vi "step_HAPS_Compressor.vi"(8 "error in":errorcluster) -> (0 "error out":errorcluster)   [LabVIEW 2020]
uses:
  <vilib>/AKKA/PROVEtech-RBS/PROVEtechRBS.lvlib
  <vilib>/AKKA/PROVEtech-RBS/SubVIs/Write (Signals Single-point).vi
  <vilib>/AKKA/PROVEtech-RBS/SubVIs/Read (Signals Single-point).vi
panel:
  out "receive unit":string[](array[string])
  out "pass":bool
  out "Array out":string[](array[string])
  out "receive signals":string[](array[string])
  out "sgl array":dbl[](array[numeric])
  out "send unit":string[](array[string])
  out "send values":string[](array[string])
  out "send signals":string[](array[string])
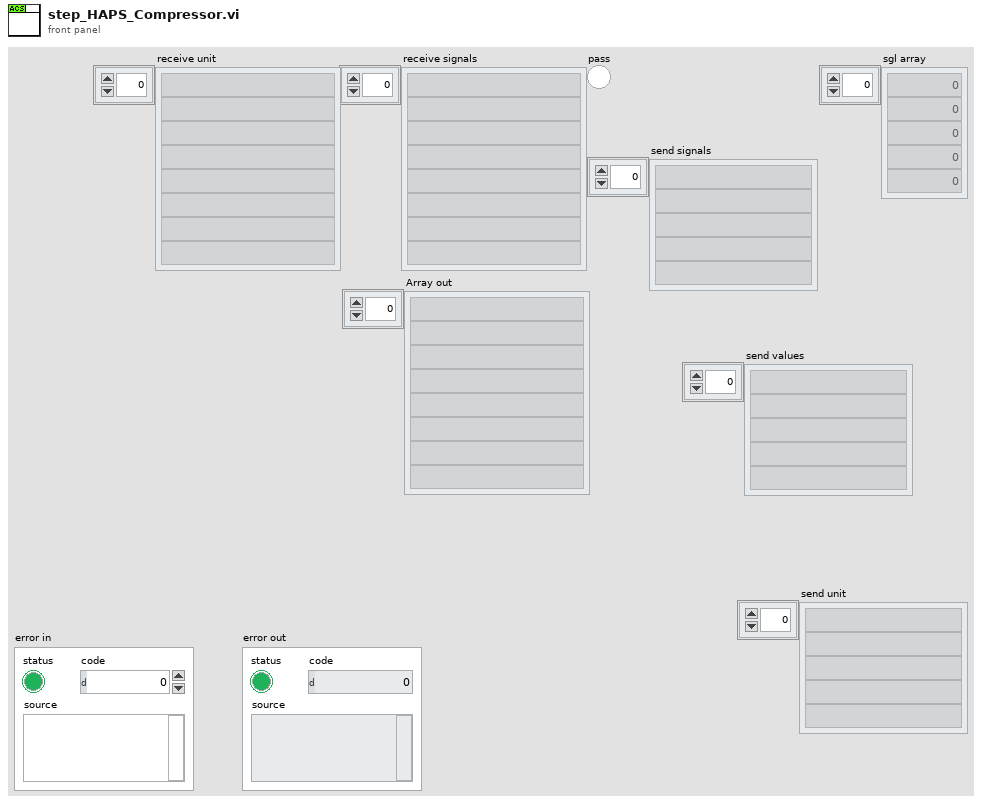
[diagram p1: front panel]
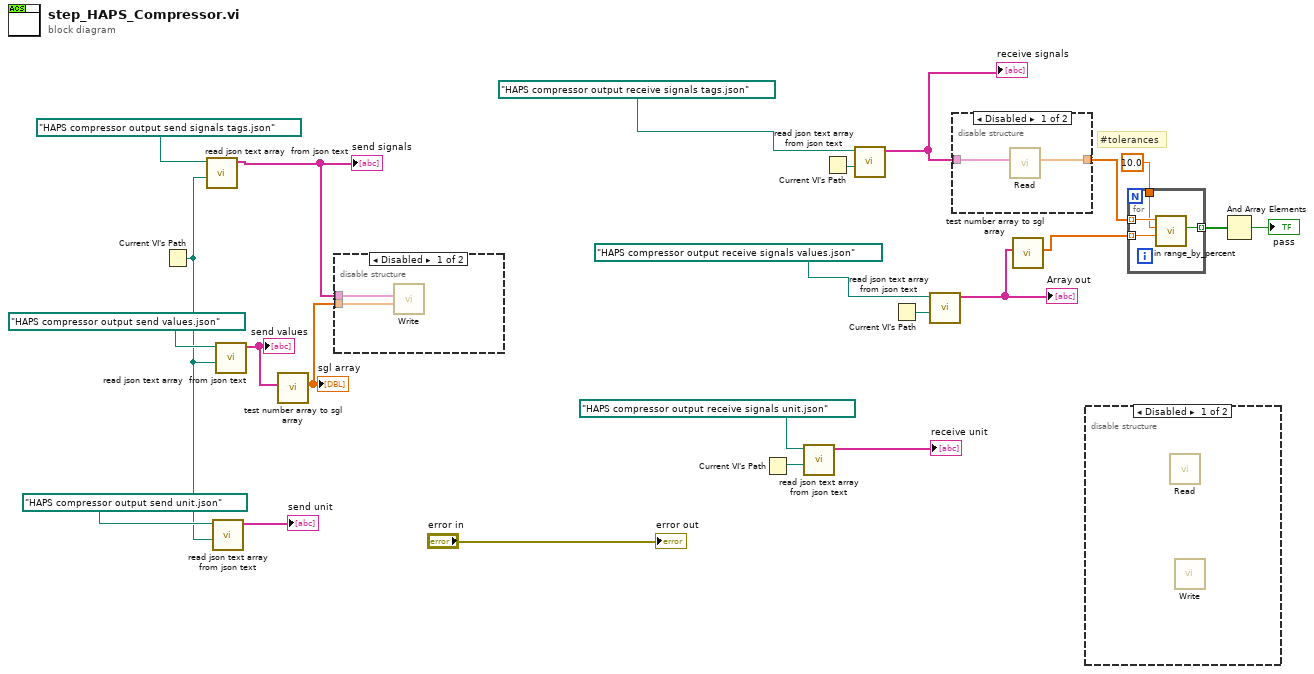
[diagram p0: block diagram]
diagram:
  # "#tolerances"
  n1 = Current VI's Path() -> (path=w19:path)
  n2 = call "read json text array  from json text.vi"("this vis path"=w19, "file name"=path "HAPS compressor output send signals tags.json" ("name or relative path")) -> ("Array out"=w17:string[])  [unwired: 8 in, 1 out]
  "send signals" <- w17
  n3 = call "read json text array  from json text.vi"("this vis path"=w19, "file name"=path "HAPS compressor output send unit.json" ("name or relative path")) -> ("Array out"=→"send unit":string[])  [unwired: 8 in, 1 out]
  n4 = call "read json text array  from json text.vi"("this vis path"=w19, "file name"=path "HAPS compressor output send values.json" ("name or relative path")) -> ("Array out"=w18:string[])  [unwired: 8 in, 1 out]
  "send values" <- w18
  n5 = call "test number array to sgl array.vi"("send values"=w18) -> ("sgl array"=w16:dbl[])  [unwired: 10 in]
  "sgl array" <- w16
  n6 = disable-structure shown="Disabled" {
    disable-tunnel: w17 -> [w25 _]
    disable-tunnel: w16 -> [w24 _]
    frame Disabled {
      n7 = call-poly <vilib>:"Write.vi"("values"=w24, "signals"=w25) -> ()  [unwired: 8 in, 2 out]
    }
    frame Enabled {
    }
  }
  n8 = Current VI's Path() -> (path=w4:path)
  n9 = call "read json text array  from json text.vi"("this vis path"=w4, "file name"=path "HAPS compressor output receive signals unit.json" ("name or relative path")) -> ("Array out"=→"receive unit":string[])  [unwired: 8 in, 1 out]
  n10 = Current VI's Path() -> (path=w14:path)
  n11 = call "read json text array  from json text.vi"("this vis path"=w14, "file name"=path "HAPS compressor output receive signals tags.json" ("name or relative path")) -> ("Array out"=w10:string[])  [unwired: 8 in, 1 out]
  "receive signals" <- w10
  n12 = Current VI's Path() -> (path=w12:path)
  n13 = call "read json text array  from json text.vi"("this vis path"=w12, "file name"=path "HAPS compressor output receive signals values.json" ("name or relative path")) -> ("Array out"=w11:string[])  [unwired: 8 in, 1 out]
  "Array out" <- w11
  n14 = disable-structure shown="Disabled" {
    disable-tunnel: w10 -> [w27 _]
    disable-tunnel: [w26 _] -> w9
    frame Disabled {
      n15 = call-poly <vilib>:"Read.vi"("signals"=w27) -> ("values"=w26:dbl[])  [unwired: 8 in, 2 out]
    }
    frame Enabled {
    }
  }
  n16 = call "test number array to sgl array.vi"("send values"=w11) -> ("sgl array"=w8:dbl[])  [unwired: 10 in]
  n17 = disable-structure shown="Disabled" {
    frame Disabled {
      n18 = call-poly <vilib>:"Read.vi"() -> ()  [unwired: 9 in, 3 out]
      n19 = call-poly <vilib>:"Write.vi"() -> ()  [unwired: 10 in, 2 out]
    }
    frame Enabled {
    }
  }
  n20 = for {
    tunnel: w9 -> [w31] mode=indexing
    tunnel: w8 -> [w30] mode=indexing
    tunnel: 10.0 ("tol %") -> [w29]
    tunnel: [w28] -> w6 mode=indexing
    n21 = call "in range_by_percent.vi"("setpoint"=w30, "tol %"=w29, "x"=w31) -> ("In Range?"=w28:bool)  [unwired: 5 in, 3 out]
  }
  n22 = And Array Elements(Boolean array=w6) -> (logical AND=→"pass":bool)
  "error out" <- "error in"
